vi "Untitled 1.vi"() -> ()   [LabVIEW 2017]
panel:
  out "Array":string[](array[string])
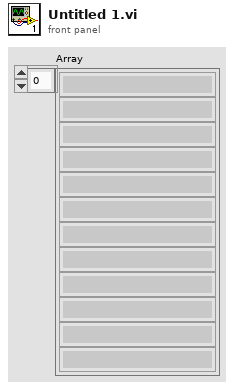
[diagram p1: front panel]
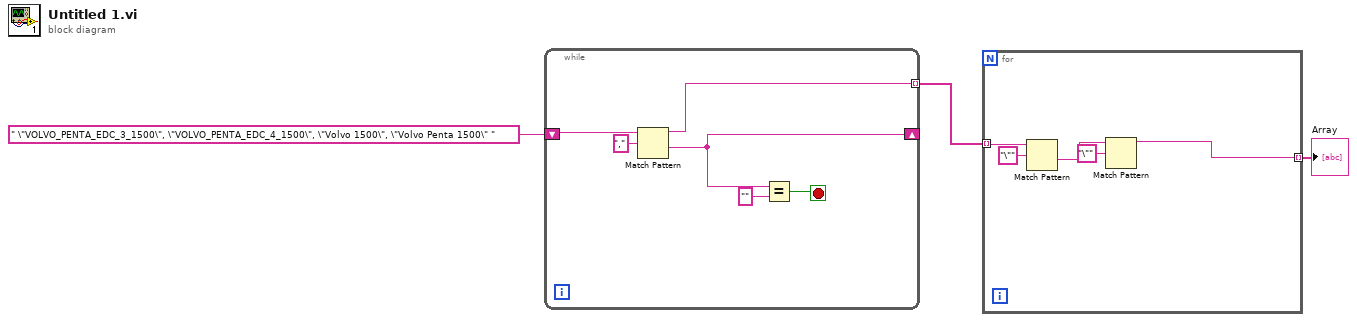
[diagram p0: block diagram]
diagram:
  n1 = while {
    shift-right: [w6] -> _
    shift-left: " \"VOLVO_PENTA_EDC_3_1500\", \"VOLVO_PENTA_EDC_4_1500\", \"Volvo 1500\", \"Volvo Penta 1500\" " -> [w9]
    tunnel: [w7] -> w2 mode=indexing
    stop <- w4 stop-if-true
    n2 = Match Pattern(string=w9, regular expression=",") -> (before substring=w7:string, after substring=w6:string)  [unwired: 1 in, 2 out]
    n3 = Equal?(x=w6, y="") -> (x = y?=w4:bool)
  }
  n4 = for {
    tunnel: w2 -> [w14] mode=indexing
    tunnel: [w10] -> w1 mode=indexing
    n5 = Match Pattern(string=w14, regular expression="\"") -> (after substring=w12:string)  [unwired: 1 in, 3 out]
    n6 = Match Pattern(string=w12, regular expression="\"") -> (before substring=w10:string)  [unwired: 1 in, 3 out]
  }
  "Array" <- w1
